vi "Set A Bit U8.vi"(9 "Input":u8 format="%08x", 10 "B":bool, 11 "Bit Number":u8) -> (3 "Output":u8 format="%08x")   [LabVIEW 2024]
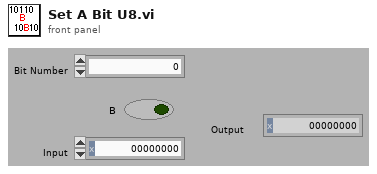
[diagram p1: front panel]
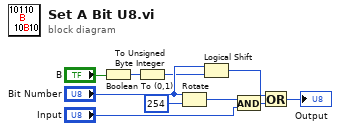
[diagram p0: block diagram]
diagram:
  n1 = Boolean To (0,1)(Boolean="B") -> (0, 1=w6:i16)
  n2 = To Unsigned Byte Integer(number=w6) -> (unsigned 8bit integer=w2:u8)
  n3 = Rotate(1:u8 254 ("x"), 2:"Bit Number") -> (0:w1:u8)
  n4 = Logical Shift(y="Bit Number", x=w2) -> (x << y=w3:u8)
  n5 = And(x=w1, y="Input") -> (x .and. y?=w8:u8)
  n6 = Or(x=w3, y=w8) -> (x .or. y?=→"Output":u8)
